vi "UpdateParenthood.vi"(8 "error in (no error)":errorcluster, 11 "GenLVOOP in":refnum<class "GenLVOOP.lvclass">) -> (0 "error out":errorcluster, 3 "GenLVOOP out":refnum<class "GenLVOOP.lvclass">)   [LabVIEW 2013, in "GenLVOOP.lvclass"]
uses:
  GenLVOOP.lvclass
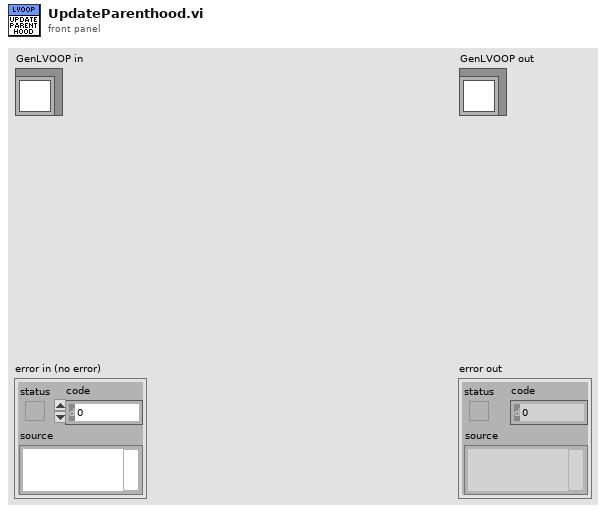
[diagram p1: front panel]
types:
  T1 = typedef "baseClass.lvclass/propertyDef.ctl" = cluster{"Name":string, "types":T2, "UserDefined":string, "Array":bool}
  T2 = typedef "baseClass.lvclass/types.ctl" = enum16{"string", "int", "decimal", "bool", "class", "enum"}
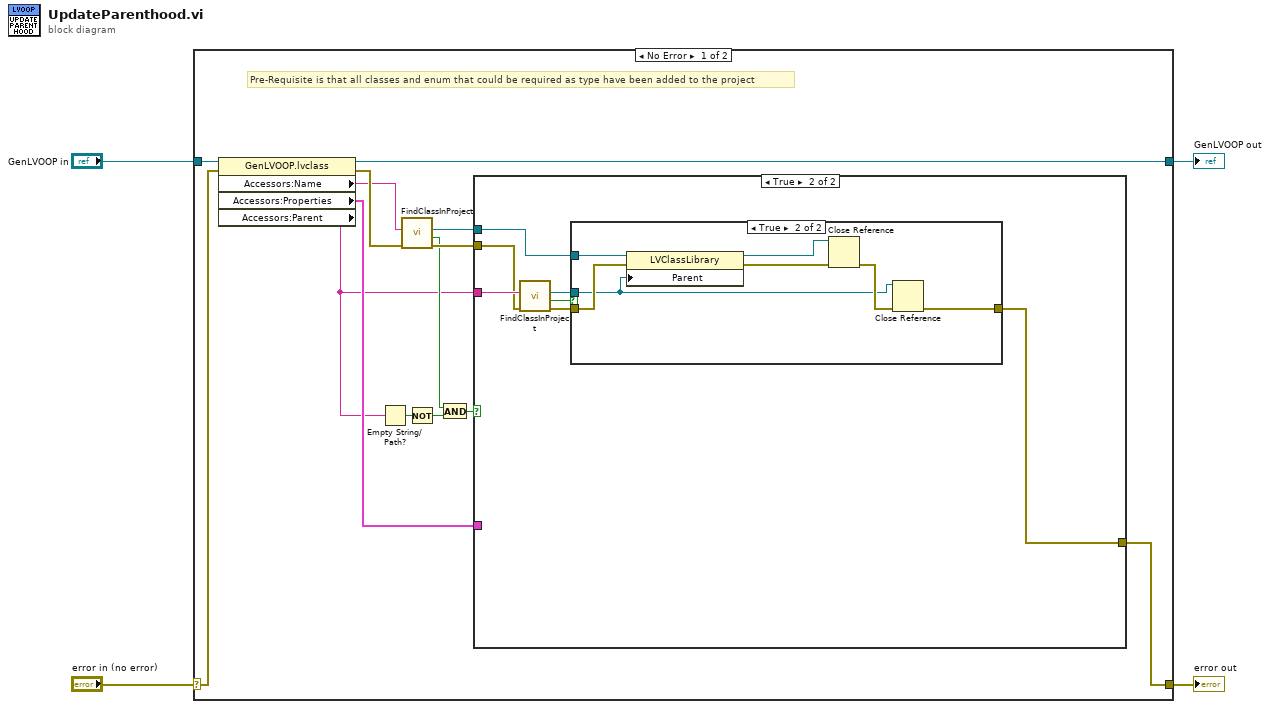
[diagram p0: block diagram]
diagram:
  n1 = case shown="No Error" "error in (no error)" {
    selector: "error in (no error)" -> [w16 w36]
    tunnel: [w17 w36] -> w3
    tunnel: [w12 w35] -> w1
    tunnel: "GenLVOOP in" -> [w18 w35]
    frame No Error {
      # "Pre-Requisite is that all classes and enum that could be required as type have been added to the project"
      n2 = property class="GenLVOOP.lvclass"(reference=w18, error in=w16) -> (reference out=w12:refnum<class "GenLVOOP.lvclass">, error out=w14:errorcluster, "Accessors:Name"=w10:string, "Accessors:Properties"=w11:T1[], "Accessors:Parent"=w5:string)
      n3 = Empty String/Path?(string/path=w5) -> (empty?=w6:bool)
      n4 = call "FindClassInProject.vi"("error in (no error)"=w14, "Name"=w10) -> ("error out"=w13:errorcluster, "Found"=w8:bool, "LVClassLibrary Refnum"=w15:refnum<vi>)  [unwired: 7 in]
      n5 = Not(x=w6) -> (.not. x?=w7:bool)
      n6 = And(x=w8, y=w7) -> (x .and. y?=w9:bool)
      n7 = case shown="True" w9 {
        tunnel: [w19 w20] -> w17
        tunnel: w15 -> [_ w24]
        tunnel: w13 -> [w19 w25]
        tunnel: w11 -> [_ _]
        tunnel: w5 -> [_ w26]
        frame False {
        }
        frame True {
          n8 = call "FindClassInProject.vi"("error in (no error)"=w25, "Name"=w26) -> ("error out"=w21:errorcluster, "Found"=w22:bool, "LVClassLibrary Refnum"=w23:refnum<vi>)  [unwired: 7 in]
          n9 = case shown="True" w22 {
            tunnel: w24 -> [_ w34]
            tunnel: w23 -> [_ w29]
            tunnel: w21 -> [w27 w33]
            tunnel: [w27 w28] -> w20
            frame False {
            }
            frame True {
              n10 = property class="LVClassLibrary"(reference=w34, error in=w33, "Parent"=w29) -> (reference out=w31:refnum<vi>, error out=w32:errorcluster)
              n11 = Close Reference(reference=w31, error in (no error)=w32) -> (error out=w30:errorcluster)
              n12 = Close Reference(reference=w29, error in (no error)=w30) -> (error out=w28:errorcluster)
            }
          }
        }
      }
    }
    frame Error {
    }
  }
  "error out" <- w3
  "GenLVOOP out" <- w1
